vi "Plugin Configuration.Method.Get Resource URL.vi"(8 "error in (no error)":errorcluster, 11 "Plugin Model in":refnum<class "Plugin Configuration.lvclass">) -> (0 "error out":errorcluster, 2 "resource url":string, 3 "Plugin Model out":refnum<class "Plugin Configuration.lvclass">)   [LabVIEW 2016, in "Plugin Configuration.lvclass"]
uses:
  Plugin Configuration.lvclass
  Plugin Configuration.lvclass/Plugin Configuration.ctl
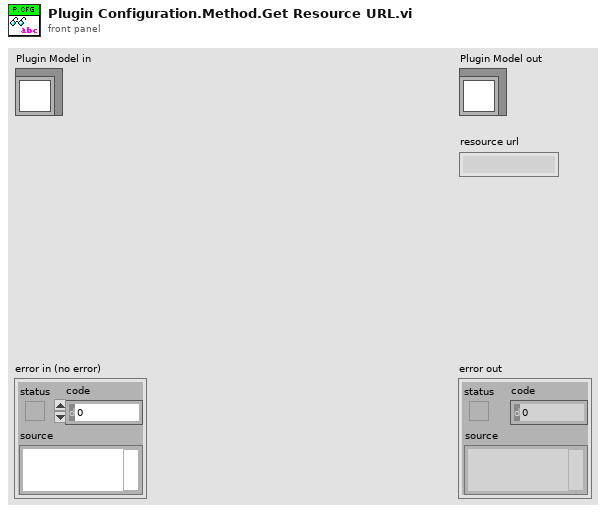
[diagram p1: front panel]
types:
  T1 = typedef "Plugin Configuration.lvclass/Plugin Configuration.Typedef.URL Configuration.ctl" = cluster{"protocol":string, "body":string}
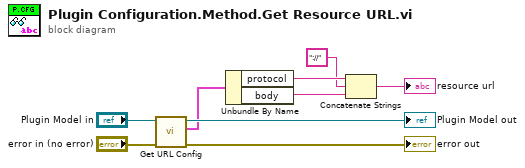
[diagram p0: block diagram]
diagram:
  n1 = call "Get URL Config.vi"("error in (no error)"="error in (no error)", "Plugin Model in"="Plugin Model in") -> ("error out"=→"error out":errorcluster, "url config"=w5:T1, "Plugin Model out"=→"Plugin Model out":refnum<class "Plugin Configuration.lvclass">)  [unwired: 7 in]
  n2 = Unbundle By Name(w5) -> ("protocol"=w4:string, "body"=w1:string)
  n3 = Concatenate Strings(w4, "://", w1) -> (→"resource url":string)
